vi "Initialise.vi"(8 "error in (no error)":errorcluster, 10 "Data Rate (12.5Hz)":T1=enum."12.5Hz", 11 "HTS221 in":refnum<class "HTS221.lvclass">) -> (0 "error out":errorcluster, 3 "HTS221 out":refnum<class "HTS221.lvclass">)   [LabVIEW 2020, in "HTS221.lvclass"]
doc: "Reads the calibration values and initialises the HTS221."
uses:
  HTS221.lvclass
  HTS221 Data Rates.ctl
  LINX I2C/LINX I2C.lvclass
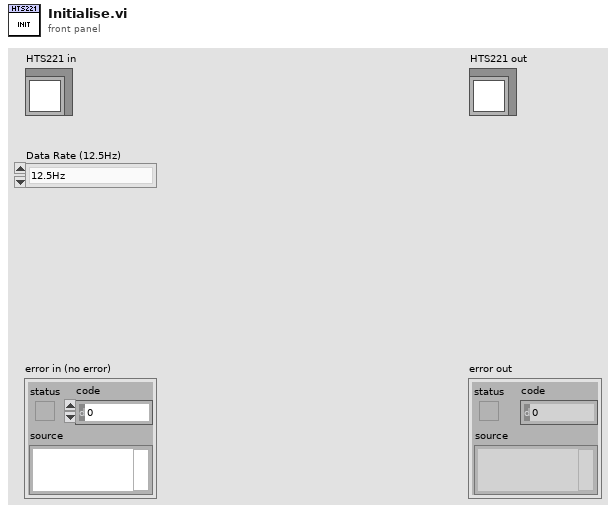
[diagram p1: front panel]
types:
  T1 = typedef "HTS221.lvclass/HTS221 Data Rates.ctl" = enum16{"One-Shot", "1Hz", "7Hz", "12.5Hz"}
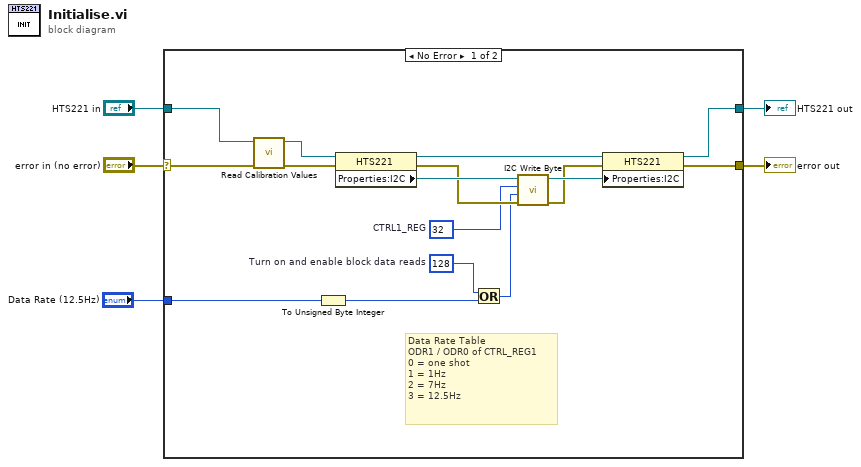
[diagram p0: block diagram]
diagram:
  n1 = case shown="No Error" "error in (no error)" {
    selector: "error in (no error)" -> [w20 w23]
    tunnel: [w12 w23] -> w4
    tunnel: [w11 w22] -> w2
    tunnel: "HTS221 in" -> [w21 w22]
    tunnel: "Data Rate (12.5Hz)" -> [w8 _]
    frame No Error {
      w9 = u8 128  # Turn on and enable block data reads
      w15 = u8 32  # CTRL1_REG
      # "Data Rate Table\nODR1 / ODR0 of CTRL_REG1\n0 = one shot\n1 = 1Hz\n2 = 7Hz\n3 = 12.5Hz"
      n2 = call "Read Calibration Values.vi"("error in (no error)"=w20, "HTS221 in"=w21) -> ("error out"=w19:errorcluster, "HTS221 out"=w18:refnum<class "HTS221.lvclass">)  [unwired: 8 in]
      n3 = To Unsigned Byte Integer(number=w8) -> (unsigned 8bit integer=w6:u8)
      n4 = property class="HTS221"(reference=w18, error in=w19) -> (reference out=w10:refnum<class "HTS221.lvclass">, error out=w16:errorcluster, "Properties:I2C"=w17:refnum<class "LINX I2C.lvclass">)
      n5 = Or(x=w9, y=w6) -> (x .or. y?=w7:u8)
      n6 = call "I2C Write Byte.vi"("error in (no error)"=w16, "Value"=w7, "Register Address"=w15, "LINX I2C in"=w17) -> ("error out"=w13:errorcluster, "LINX I2C out"=w14:refnum<class "LINX I2C.lvclass">)  [unwired: 6 in]
      n7 = property class="HTS221"(reference=w10, error in=w13, "Properties:I2C"=w14) -> (reference out=w11:refnum<class "HTS221.lvclass">, error out=w12:errorcluster)
    }
    frame Error {
    }
  }
  "error out" <- w4
  "HTS221 out" <- w2
